vi "Write Boolean.vi"() -> ()   [LabVIEW 2012, in "configlib.lvlib"]
uses:
  configlib.lvlib
  Configuration File Definition.ctl
  File Options.ctl
panel:
  out "Configuration Reference Out":refnum<data-value>
  in  "Configuration Reference In":refnum<data-value>
  out "found?":bool
  in  "value":bool
  in  "key":string
  in  "section":string
  out "error out":errorcluster
  in  "error in (no error)":errorcluster
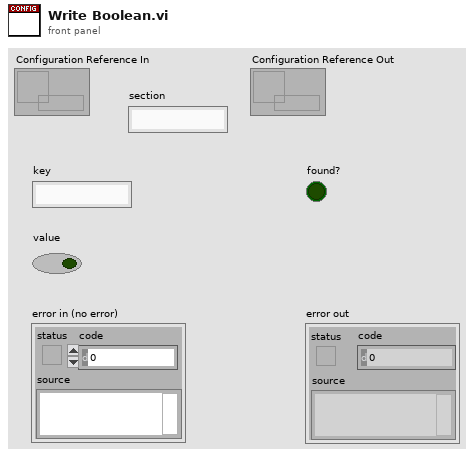
[diagram p1: front panel]
types:
  T1 = typedef "configlib.lvlib/Configuration File Definition.ctl" = cluster{"dirty":bool, "path":path, "Fileopts":T2, "Section Lookup":variant, "Key Lookup":variant, "Raw File":string[]}
  T2 = typedef "configlib.lvlib/File Options.ctl" = cluster{"Name/Value delimiter (\"=\")":string, "Comment delimiter (\";\")":string}
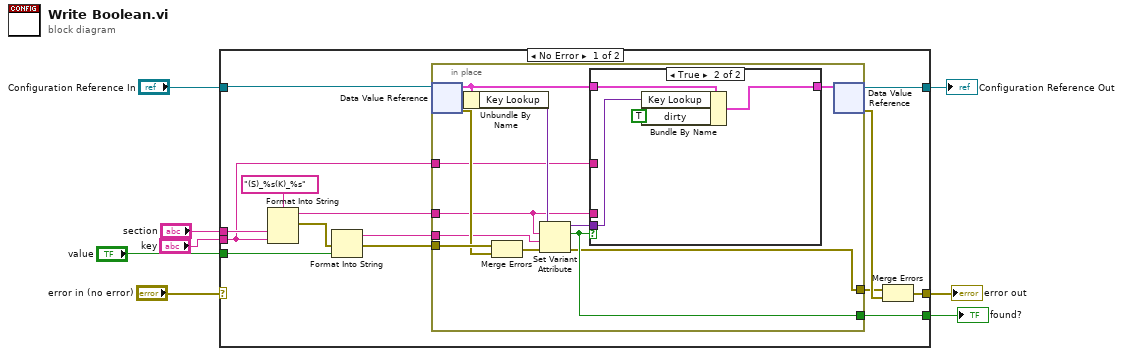
[diagram p0: block diagram]
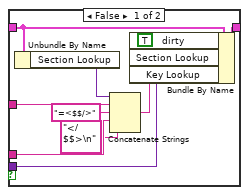
[diagram p2: hidden frame]
diagram:
  n1 = case shown="No Error" "error in (no error)" {
    selector: "error in (no error)" -> [_ w50]
    tunnel: [w15 w50] -> w7
    tunnel: "Configuration Reference In" -> [w17 w49]
    tunnel: [w16 w49] -> w5
    tunnel: "value" -> [w22 _]
    tunnel: "section" -> [w20 _]
    tunnel: "key" -> [w10 _]
    tunnel: [w11 _] -> w1
    frame No Error {
      n2 = Format Into String(format string="(S)_%s(K)_%s", w20, w10) -> (resulting string=w13:string, error out=w21:errorcluster)  [unwired: 2 in]
      n3 = Format Into String(error in=w21, w22) -> (resulting string=w12:string, error out=w18:errorcluster)  [unwired: 2 in]
      n4 = in-place {
        in-place-border: w18 -> [w34]
        in-place-border: w13 -> [w24]
        in-place-border: w12 -> [w27]
        in-place-border: [w26] -> w11
        in-place-border: w10 -> [w25]
        in-place-border: [w23] -> w9
        n5 = in-place-dvr #1(w17) -> (w29:T1, w33:errorcluster)
        n6 = Unbundle By Name(w29) -> ("Key Lookup"=w31:variant)
        n7 = Merge Errors(w34, w33) -> (w32:errorcluster)
        n8 = Set Variant Attribute(Variant=w31, name=w24, value=w27, error in=w32) -> (Variant out=w30:variant, replaced=w26:bool, error out=w23:errorcluster)
        n9 = case shown="True" w26 {
          tunnel: w30 -> [w42 w47]
          tunnel: w29 -> [w44 w48]
          tunnel: [w43 w46] -> w28
          tunnel: w25 -> [w38 _]
          tunnel: w24 -> [w36 _]
          frame False {
            n10 = Unbundle By Name(w44) -> ("Section Lookup"=w40:variant)
            n11 = Concatenate Strings(w40, w38, "=<$$/>" ("string"), w36, "</$$>\n" ("string")) -> (w39:string)
            n12 = Bundle By Name(cluster=w44, "dirty"=TRUE, "Section Lookup"=w39, "Key Lookup"=w42) -> (w43:T1)
          }
          frame True {
            n13 = Bundle By Name(cluster=w48, "Key Lookup"=w47, "dirty"=TRUE) -> (w46:T1)
          }
        }
        n14 = in-place-dvr #1(w28) -> (w16:refnum<data-value>, w14:errorcluster)
      }
      n15 = Merge Errors(w9, w14) -> (w15:errorcluster)
    }
    frame Error {
    }
  }
  "Configuration Reference Out" <- w5
  "error out" <- w7
  "found?" <- w1
